vi "Count Start.vi"(8 "error in (no error)":errorcluster, 10 "Trigger Mode":u32(ring), 11 "Handle":u32) -> (0 "error out":errorcluster, 3 "Status":i32)   [LabVIEW 2014, in "Photon Counter.lvlib" / "C8855-01.lvlib"]
doc: "This unit starts counting using the trigger type specified by TriggerMode.\n\n\nBOOL C8855API __stdcall C8855CountStart( HANDLE hC8855,\n BYTE TriggerMode );"
uses:
  C8855-01.lvlib
  C8855-01api.dll
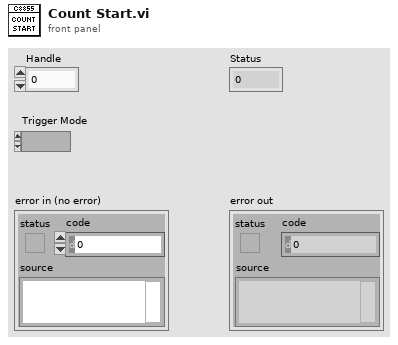
[diagram p1: front panel]
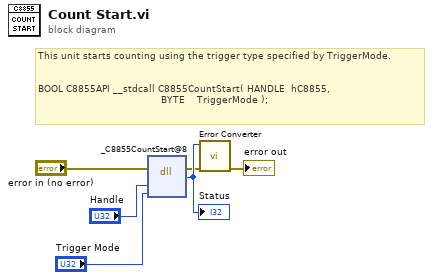
[diagram p0: block diagram]
diagram:
  # "This unit starts counting using the trigger type specified by TriggerMode.\n\n\nBOOL C8855API __stdcall C8855CountStart( HANDLE  hC8855,\n                                         BYTE    TriggerMode );"
  n1 = dll-call lib="C:/Users/Andy/Desktop/Trace Grabber/Drivers/C8855-01/C8855-01api.dll" fn="_C8855CountStart@8"(error in="error in (no error)", "Handle"="Handle", "Trigger Mode"="Trigger Mode") -> (error out=w2:errorcluster, "return type"=w6:i32)  [unwired: 4 in, 1 out]
  "Status" <- w6
  n2 = call "Error Converter.vi"("error in (no error)"=w2, "error code"=w6) -> ("error out"=→"error out":errorcluster)  [unwired: 9 in]
